vi "Build Tree from Section Change List.vi"(8 "error in (no error)":errorcluster, 9 "Database Changes":T1 {"Missing"."Node Ref" format="%.0x"; "Changed"."Old"."Node Ref" format="%.0x"}, 10 "Section":string="Incoming", 11 "TreeControl in":refnum<vi>) -> (0 "error out":errorcluster, 3 "TreeControl out":refnum<vi>)   [LabVIEW 2025, in "Protection and Counter Addon System Explorer.lvlib"]
uses:
  Protection and Counter Addon System Explorer.lvlib
  Types/Database Changes.ctl
  Types/Base Frame Info_NoVS.ctl
  Types/Signal Attributes.ctl
  Types/CAN Filter Type.ctl
  Types/Base Frame Info.ctl
  <vilib>/NI VeriStand/Custom Device API/Custom Device Item Ref.ctl
  Types/Related CAN Frames.ctl
  Types/Related CAN Frames No VS.ctl
  Types/Tree Item Settings.ctl
  <vilib>/NI VeriStand/Custom Device API/Custom Device API.lvlib
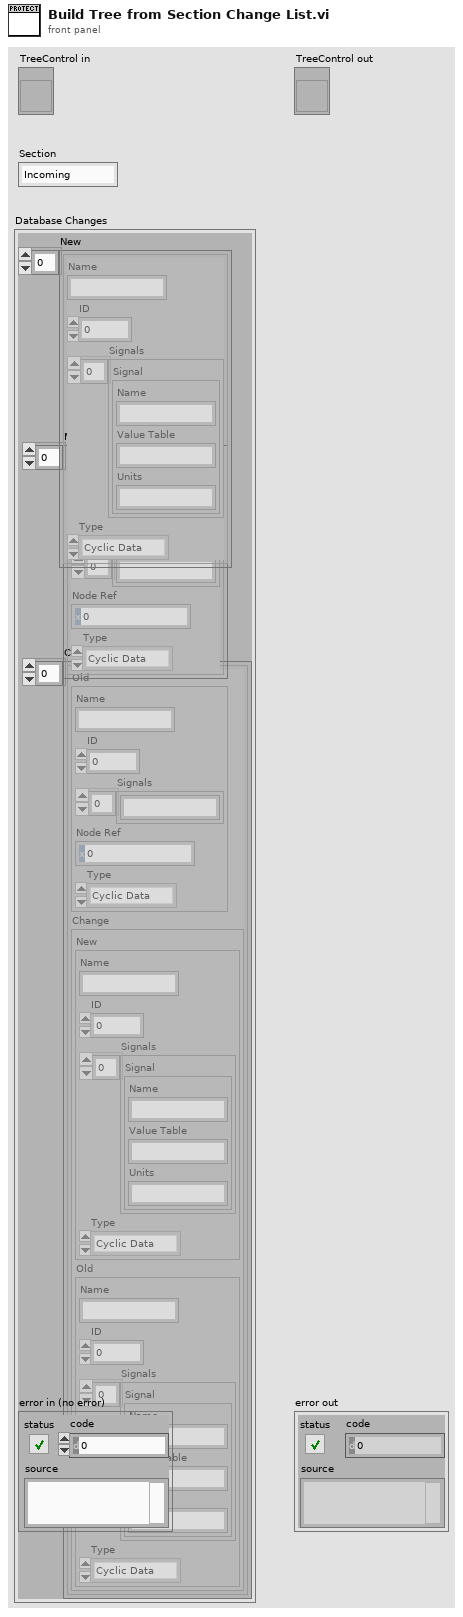
[diagram p1: front panel]
types:
  T1 = typedef "Protection and Counter Addon System Explorer.lvlib/Database Changes.ctl" = cluster{"New":T2[], "Missing":T5[], "Changed":T7[]}
  T2 = typedef "Protection and Counter Addon System Explorer.lvlib/Base Frame Info_NoVS.ctl" = cluster{"Name":string, "ID":u32, "Signals":T3[], "Type":T4}
  T3 = typedef "Protection and Counter Addon System Explorer.lvlib/Signal Attributes.ctl" = cluster{"Name":string, "Value Table":string, "Units":string}
  T4 = typedef "Protection and Counter Addon System Explorer.lvlib/CAN Filter Type.ctl" = enum16{"Cyclic Data", "Event Data", "Cyclic/Event", "All"}
  T5 = typedef "Protection and Counter Addon System Explorer.lvlib/Base Frame Info.ctl" = cluster{"Name":string, "ID":u32, "Signals":string[], "Node Ref":T6, "Type":T4}
  T6 = typedef "Custom Device API.lvlib/Custom Device Item Ref.ctl" = u64
  T7 = typedef "Protection and Counter Addon System Explorer.lvlib/Related CAN Frames.ctl" = cluster{"Old":T5, "Change":T8}
  T8 = typedef "Protection and Counter Addon System Explorer.lvlib/Related CAN Frames No VS.ctl" = cluster{"New":T2, "Old":T2}
  T9 = typedef "Protection and Counter Addon System Explorer.lvlib/Tree Item Settings.ctl" = cluster{"Name":string, "Background Color":u32, "Symbol":i32, "ChildText":string, "Disable":bool}
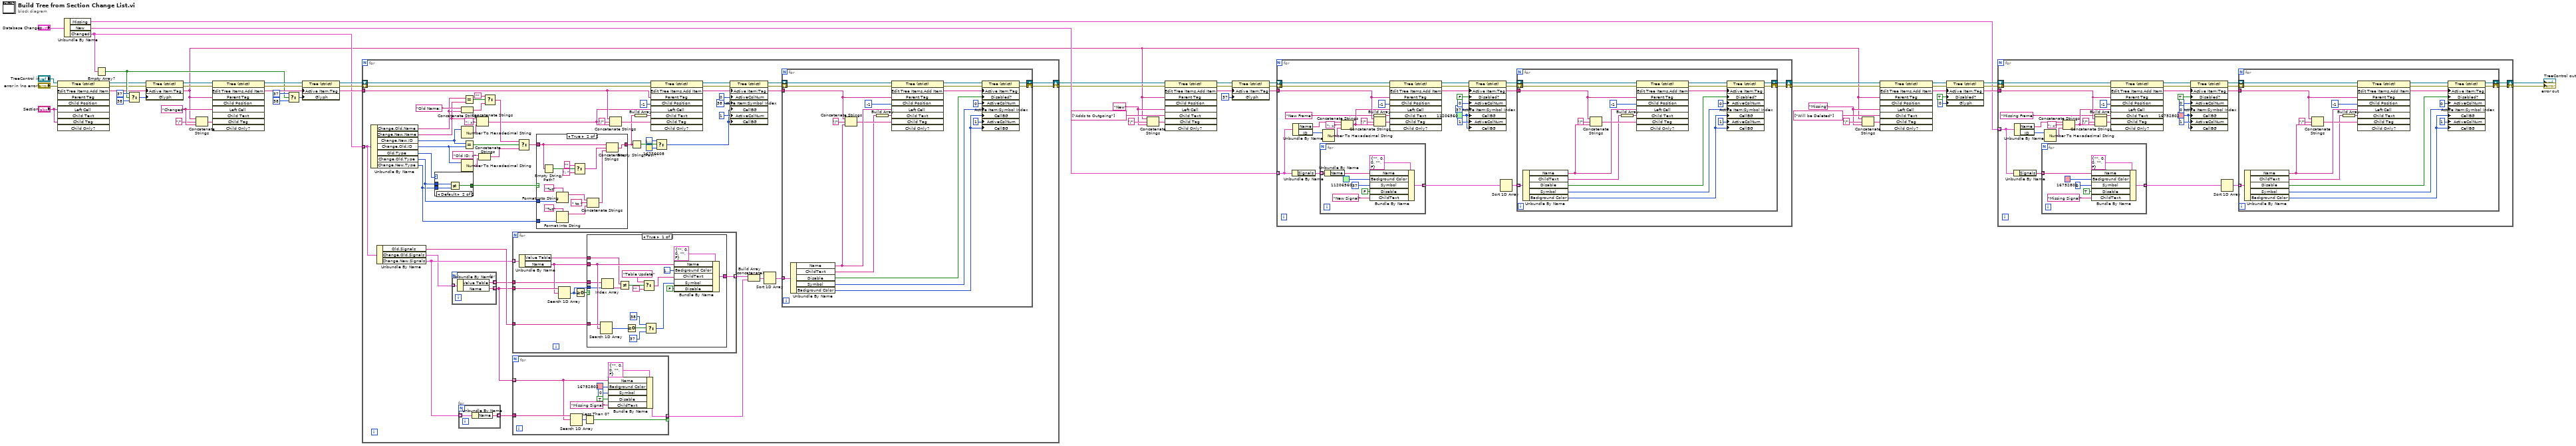
[diagram p0: block diagram]
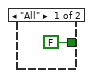
[diagram p2: hidden frame]
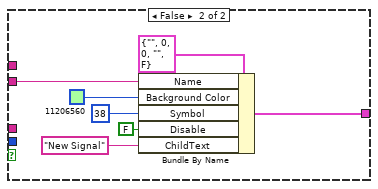
[diagram p4: hidden frame]
diagram:
  w3 = "Missing" ("Parent Tag")
  w6 = "New" ("Parent Tag")
  w22 = "Changed" ("Parent Tag")
  n1 = invoke on="Invoke Node" class="Tree (strict)" method="Edit Tree Items.Add Item"(reference="TreeControl in", error in="error in (no error)", "Left Cell"="Section", "Child Tag"="Section") -> (reference out=w11:refnum<vi>, error out=w9:errorcluster, "Edit Tree Items:Add Item"=w2:string)  [unwired: 5 in, 6 out]
  n2 = Unbundle By Name("Database Changes") -> ("Missing"=w35:T5[], "New"=w30:T2[], "Changed"=w19:T7[])
  n3 = Empty Array?(array=w19) -> (empty?=w12:bool)
  n4 = Select(t=37 ("Active Item:Symbol Index"), s=w12, f=38 ("Active Item:Symbol Index")) -> (s? t:f=w14:i32)
  n5 = property class="Tree (strict)"(reference=w11, error in=w9, "Active Item:Tag"=w2, "Glyph"=w14) -> (reference out=w10:refnum<vi>, error out=w8:errorcluster)
  n6 = Concatenate Strings(w2, "/" ("string"), w22) -> (w20:string)
  n7 = invoke on="Invoke Node" class="Tree (strict)" method="Edit Tree Items.Add Item"(reference=w10, error in=w8, "Parent Tag"=w2, "Left Cell"=w22, "Child Tag"=w20) -> (reference out=w37:refnum<vi>, error out=w38:errorcluster, "Edit Tree Items:Add Item"=w41:string)  [unwired: 4 in, 6 out]
  n8 = Select(t=37 ("Active Item:Symbol Index"), s=w12, f=38 ("Active Item:Symbol Index")) -> (s? t:f=w17:i32)
  n9 = property class="Tree (strict)"(reference=w37, error in=w38, "Active Item:Tag"=w41, "Glyph"=w17) -> (reference out=w40:refnum<vi>, error out=w39:errorcluster)
  n10 = for {
    tunnel: w19 -> [w80] mode=indexing
    shift-right: [w72] -> w28
    shift-left: w39 -> [w89]
    shift-right: [w71] -> w29
    shift-left: w40 -> [w105]
    tunnel: w41 -> [w68]
    n11 = Unbundle By Name(w80) -> ("Change.Old.Name"=w95:string, "Change.New.Name"=w99:string, "Change.New.ID"=w97:u32, "Change.Old.ID"=w101:u32, "Old.Type"=w60:T4, "Change.Old.Type"=w65:T4, "Change.New.Type"=w61:T4)
    n12 = Unbundle By Name(w80) -> ("Old.Signals"=w79:string[], "Change.Old.Signals"=w55:T3[], "Change.New.Signals"=w58:T3[])
    n13 = case shown="Default" w60 {
      tunnel: w65 -> [_ w117]
      tunnel: [FALSE w116] -> w64
      tunnel: w61 -> [_ w115]
      frame "All" {
      }
      frame Default {
        n14 = Not Equal?(x=w117, y=w115) -> (x != y?=w116:bool)
      }
    }
    n15 = for {
      tunnel: w55 -> [w111] mode=indexing
      tunnel: [w110] -> w59 mode=indexing
      tunnel: [w109] -> w56 mode=indexing
      n16 = Unbundle By Name(w111) -> ("Value Table"=w109:string, "Name"=w110:string)
    }
    n17 = for {
      tunnel: w58 -> [w113] mode=indexing
      tunnel: [w112] -> w57 mode=indexing
      n18 = Unbundle By Name(w113) -> ("Name"=w112:string)
    }
    n19 = Concatenate Strings("Old Name: ", w95) -> (w90:string)
    n20 = Number To Hexadecimal String(2:w97) -> (0:w96:string)  [unwired: 1 in]
    n21 = Number To Hexadecimal String(2:w101) -> (0:w100:string)  [unwired: 1 in]
    n22 = Equal?(x=w95, y=w99) -> (x = y?=w91:bool)
    n23 = Equal?(x=w97, y=w101) -> (x = y?=w94:bool)
    n24 = Concatenate Strings(w99, ": x" ("string"), w96) -> (w67:string)
    n25 = Concatenate Strings("Old ID: x", w100) -> (w93:string)
    n26 = Select(t="", s=w91, f=w90) -> (s? t:f=w87:string)
    n27 = for {
      tunnel: w59 -> [w171]
      tunnel: w58 -> [w169] mode=indexing
      tunnel: [w170] -> w78 mode=indexing
      tunnel: w79 -> [w166]
      tunnel: w56 -> [w163]
      n28 = Unbundle By Name(w169) -> ("Value Table"=w165:string, "Name"=w167:string)
      n29 = Search 1D Array(1D array=w171, element=w167) -> (index of element=w164:i32)  [unwired: 1 in]
      n30 = Greater Or Equal To 0?(x=w164) -> (x >= 0?=w168:bool)
      n31 = case shown="True" w168 {
        tunnel: [w184 w195] -> w170
        tunnel: w167 -> [w180 w191]
        tunnel: w166 -> [w182 _]
        tunnel: w165 -> [w176 _]
        tunnel: w164 -> [w178 _]
        tunnel: w163 -> [w179 _]
        frame True {
          n32 = Search 1D Array(1D array=w182, element=w180) -> (index of element=w183:i32)  [unwired: 1 in]
          n33 = Index Array(array=w179, index=w178) -> (element=w177:string)
          n34 = Not Equal?(x=w176, y=w177) -> (x != y?=w175:bool)
          n35 = Greater Or Equal To 0?(x=w183) -> (x >= 0?=w181:bool)
          n36 = Select(t="Table Update", s=w175, f="") -> (s? t:f=w172:string)
          n37 = Select(t=38 ("Active Item:Symbol Index"), s=w181, f=37 ("Active Item:Symbol Index")) -> (s? t:f=w187:i32)
          n38 = Bundle By Name(cluster=T9 {"Name"="", "Background Color"=0, "Symbol"=0, "ChildText"="", "Disable"=FALSE}, "Name"=w180, "Background Color"=u32 16777216, "ChildText"=w172, "Symbol"=w187, "Disable"=FALSE) -> (w184:T9)
        }
        frame False {
          n39 = Bundle By Name(cluster=T9 {"Name"="", "Background Color"=0, "Symbol"=0, "ChildText"="", "Disable"=FALSE}, "Name"=w191, "Background Color"=u32 11206560, "Symbol"=38 ("Active Item:Symbol Index"), "Disable"=FALSE, "ChildText"="New Signal" ("string")) -> (w195:T9)
        }
      }
    }
    n40 = for {
      tunnel: w57 -> [w162]
      tunnel: w59 -> [w153] mode=indexing
      tunnel: [w157] -> w77 mode=indexing if=w160
      n41 = Search 1D Array(1D array=w162, element=w153) -> (index of element=w161:i32)  [unwired: 1 in]
      n42 = Less Than 0?(x=w161) -> (x < 0?=w160:bool)
      n43 = Bundle By Name(cluster=T9 {"Name"="", "Background Color"=0, "Symbol"=0, "ChildText"="", "Disable"=FALSE}, "Name"=w153, "Background Color"=u32 16752802, "Symbol"=0 ("Active Item:Symbol Index"), "Disable"=TRUE, "ChildText"="Missing Signal" ("string")) -> (w157:T9)
    }
    n44 = Select(t=w87, s=w94, f=w93) -> (s? t:f=w63:string)
    n45 = case shown="True" w64 {
      tunnel: w65 -> [_ w132]
      tunnel: [w118 w130] -> w62
      tunnel: w63 -> [w118 w119]
      tunnel: w61 -> [_ w124]
      frame False {
      }
      frame True {
        n46 = Empty String/Path?(string/path=w119) -> (empty?=w129:bool)
        n47 = Format Into String(format string="%s", w132) -> (resulting string=w123:string)  [unwired: 2 in, 1 out]
        n48 = Format Into String(format string="%s", w124) -> (resulting string=w121:string)  [unwired: 2 in, 1 out]
        n49 = Select(t="", s=w129, f="; ") -> (s? t:f=w127:string)
        n50 = Concatenate Strings(w123, " to " ("string"), w121) -> (w120:string)
        n51 = Concatenate Strings(w119, w127, w120) -> (w130:string)
      }
    }
    n52 = Concatenate Strings(w68, "/" ("string"), w67) -> (w66:string)
    n53 = Empty String/Path?(string/path=w62) -> (empty?=w86:bool)
    n54 = Build Array(w62) -> (w88:string[])
    n55 = invoke on="Invoke Node" class="Tree (strict)" method="Edit Tree Items.Add Item"(reference=w105, error in=w89, "Parent Tag"=w68, "Child Position"=-1, "Left Cell"=w67, "Child Text"=w88, "Child Tag"=w66) -> (reference out=w108:refnum<vi>, error out=w107:errorcluster, "Edit Tree Items:Add Item"=w70:string)  [unwired: 2 in, 6 out]
    n56 = Select(t=u32 16777216, s=w86, f=u32 16776608) -> (s? t:f=w81:u32)
    n57 = property class="Tree (strict)"(reference=w108, error in=w107, "Active Item:Tag"=w70, "ActiveColNum"=0 ("Active Cell:Active Column Number"), "Active Item:Symbol Index"=38, "CellBG"=w81, "ActiveColNum"=1 ("Active Cell:Active Column Number"), "CellBG"=w81) -> (reference out=w75:refnum<vi>, error out=w74:errorcluster)
    n58 = Build Array (concatenate)(w78, w77) -> (w76:T9[])
    n59 = Sort 1D Array(array=w76) -> (sorted array=w73:T9[])
    n60 = for {
      shift-right: [w137] -> w71
      shift-left: w75 -> [w150]
      shift-right: [w138] -> w72
      shift-left: w74 -> [w136]
      tunnel: w73 -> [w148] mode=indexing
      tunnel: w70 -> [w149]
      n61 = Unbundle By Name(w148) -> ("Name"=w147:string, "ChildText"=w135:string, "Disable"=w134:bool, "Symbol"=w139:i32, "Background Color"=w133:u32)
      n62 = Concatenate Strings(w149, "/" ("string"), w147) -> (w146:string)
      n63 = Build Array(w135) -> (w145:string[])
      n64 = invoke on="Invoke Node" class="Tree (strict)" method="Edit Tree Items.Add Item"(reference=w150, error in=w136, "Parent Tag"=w149, "Child Position"=-1, "Left Cell"=w147, "Child Text"=w145, "Child Tag"=w146) -> (reference out=w142:refnum<vi>, error out=w141:errorcluster, "Edit Tree Items:Add Item"=w140:string)  [unwired: 2 in, 6 out]
      n65 = property class="Tree (strict)"(reference=w142, error in=w141, "Active Item:Tag"=w140, "Disabled?"=w134, "ActiveColNum"=0 ("Active Cell:Active Column Number"), "Active Item:Symbol Index"=w139, "CellBG"=w133, "ActiveColNum"=1 ("Active Cell:Active Column Number"), "CellBG"=w133) -> (reference out=w137:refnum<vi>, error out=w138:errorcluster)
    }
  }
  n66 = Concatenate Strings(w2, "/" ("string"), w6) -> (w5:string)
  n67 = invoke on="Invoke Node" class="Tree (strict)" method="Edit Tree Items.Add Item"(reference=w29, error in=w28, "Parent Tag"=w2, "Left Cell"=w6, "Child Text"=string[] ["Adds to Outgoing"], "Child Tag"=w5) -> (reference out=w44:refnum<vi>, error out=w45:errorcluster, "Edit Tree Items:Add Item"=w43:string)  [unwired: 3 in, 6 out]
  n68 = property class="Tree (strict)"(reference=w44, error in=w45, "Active Item:Tag"=w43, "Glyph"=37 ("Active Item:Symbol Index")) -> (reference out=w47:refnum<vi>, error out=w46:errorcluster)
  n69 = for {
    tunnel: w30 -> [w213] mode=indexing
    shift-right: [w208] -> w32
    shift-left: w46 -> [w217]
    shift-right: [w207] -> w31
    shift-left: w47 -> [w223]
    tunnel: w43 -> [w204]
    w200 = u32 11206560
    n70 = Unbundle By Name(w213) -> ("Signals"=w212:T3[])
    n71 = Unbundle By Name(w213) -> ("Name"=w221:string, "ID"=w219:u32)
    n72 = for {
      tunnel: w212 -> [w251] mode=indexing
      tunnel: [w252] -> w199 mode=indexing
      n73 = Unbundle By Name(w251) -> ("Name"=w247:string)
      n74 = Bundle By Name(cluster=T9 {"Name"="", "Background Color"=0, "Symbol"=0, "ChildText"="", "Disable"=FALSE}, "Name"=w247, "Background Color"=u32 11206560, "Symbol"=37 ("Active Item:Symbol Index"), "Disable"=FALSE, "ChildText"="New Signal" ("string")) -> (w252:T9)
    }
    n75 = Number To Hexadecimal String(2:w219) -> (0:w218:string)  [unwired: 1 in]
    n76 = Concatenate Strings(w221, ": x" ("string"), w218) -> (w203:string)
    n77 = Build Array("New Frame" ("string")) -> (w216:string[])
    n78 = Concatenate Strings(w204, "/" ("string"), w203) -> (w202:string)
    n79 = invoke on="Invoke Node" class="Tree (strict)" method="Edit Tree Items.Add Item"(reference=w223, error in=w217, "Parent Tag"=w204, "Child Position"=-1, "Left Cell"=w203, "Child Text"=w216, "Child Tag"=w202) -> (reference out=w226:refnum<vi>, error out=w225:errorcluster, "Edit Tree Items:Add Item"=w206:string)  [unwired: 2 in, 6 out]
    n80 = property class="Tree (strict)"(reference=w226, error in=w225, "Active Item:Tag"=w206, "Disabled?"=FALSE ("Active Item:Disabled?"), "ActiveColNum"=0 ("Active Cell:Active Column Number"), "Active Item:Symbol Index"=37, "CellBG"=w200, "ActiveColNum"=1 ("Active Cell:Active Column Number"), "CellBG"=w200) -> (reference out=w211:refnum<vi>, error out=w210:errorcluster)
    n81 = Sort 1D Array(array=w199) -> (sorted array=w209:T9[])
    n82 = for {
      shift-right: [w231] -> w207
      shift-left: w211 -> [w244]
      shift-right: [w232] -> w208
      shift-left: w210 -> [w230]
      tunnel: w209 -> [w242] mode=indexing
      tunnel: w206 -> [w243]
      n83 = Unbundle By Name(w242) -> ("Name"=w241:string, "ChildText"=w229:string, "Disable"=w228:bool, "Symbol"=w233:i32, "Background Color"=w227:u32)
      n84 = Concatenate Strings(w243, "/" ("string"), w241) -> (w240:string)
      n85 = Build Array(w229) -> (w239:string[])
      n86 = invoke on="Invoke Node" class="Tree (strict)" method="Edit Tree Items.Add Item"(reference=w244, error in=w230, "Parent Tag"=w243, "Child Position"=-1, "Left Cell"=w241, "Child Text"=w239, "Child Tag"=w240) -> (reference out=w236:refnum<vi>, error out=w235:errorcluster, "Edit Tree Items:Add Item"=w234:string)  [unwired: 2 in, 6 out]
      n87 = property class="Tree (strict)"(reference=w236, error in=w235, "Active Item:Tag"=w234, "Disabled?"=w228, "ActiveColNum"=0 ("Active Cell:Active Column Number"), "Active Item:Symbol Index"=w233, "CellBG"=w227, "ActiveColNum"=1 ("Active Cell:Active Column Number"), "CellBG"=w227) -> (reference out=w231:refnum<vi>, error out=w232:errorcluster)
    }
  }
  n88 = Concatenate Strings(w2, "/" ("string"), w3) -> (w1:string)
  n89 = invoke on="Invoke Node" class="Tree (strict)" method="Edit Tree Items.Add Item"(reference=w31, error in=w32, "Parent Tag"=w2, "Left Cell"=w3, "Child Text"=string[] ["Will be Deleted"], "Child Tag"=w1) -> (reference out=w52:refnum<vi>, error out=w50:errorcluster, "Edit Tree Items:Add Item"=w54:string)  [unwired: 3 in, 6 out]
  n90 = property class="Tree (strict)"(reference=w52, error in=w50, "Active Item:Tag"=w54, "Disabled?"=TRUE ("Active Item:Disabled?"), "Glyph"=0 ("Active Item:Symbol Index")) -> (reference out=w53:refnum<vi>, error out=w51:errorcluster)
  n91 = for {
    tunnel: w35 -> [w270] mode=indexing
    shift-right: [w265] -> w34
    shift-left: w51 -> [w274]
    shift-right: [w264] -> w33
    shift-left: w53 -> [w280]
    tunnel: w54 -> [w261]
    w257 = u32 16752802
    n92 = Unbundle By Name(w270) -> ("Signals"=w269:string[])
    n93 = Unbundle By Name(w270) -> ("Name"=w278:string, "ID"=w276:u32)
    n94 = for {
      tunnel: w269 -> [w307] mode=indexing
      tunnel: [w308] -> w256 mode=indexing
      n95 = Bundle By Name(cluster=T9 {"Name"="", "Background Color"=0, "Symbol"=0, "ChildText"="", "Disable"=FALSE}, "Name"=w307, "Background Color"=u32 16752802, "Symbol"=0 ("Active Item:Symbol Index"), "Disable"=TRUE, "ChildText"="Missing Signal" ("string")) -> (w308:T9)
    }
    n96 = Number To Hexadecimal String(2:w276) -> (0:w275:string)  [unwired: 1 in]
    n97 = Concatenate Strings(w278, ": x" ("string"), w275) -> (w260:string)
    n98 = Build Array("Missing Frame" ("string")) -> (w273:string[])
    n99 = Concatenate Strings(w261, "/" ("string"), w260) -> (w259:string)
    n100 = invoke on="Invoke Node" class="Tree (strict)" method="Edit Tree Items.Add Item"(reference=w280, error in=w274, "Parent Tag"=w261, "Child Position"=-1, "Left Cell"=w260, "Child Text"=w273, "Child Tag"=w259) -> (reference out=w283:refnum<vi>, error out=w282:errorcluster, "Edit Tree Items:Add Item"=w263:string)  [unwired: 2 in, 6 out]
    n101 = property class="Tree (strict)"(reference=w283, error in=w282, "Active Item:Tag"=w263, "Disabled?"=TRUE ("Active Item:Disabled?"), "ActiveColNum"=0 ("Active Cell:Active Column Number"), "Active Item:Symbol Index"=0, "CellBG"=w257, "ActiveColNum"=1 ("Active Cell:Active Column Number"), "CellBG"=w257) -> (reference out=w268:refnum<vi>, error out=w267:errorcluster)
    n102 = Sort 1D Array(array=w256) -> (sorted array=w266:T9[])
    n103 = for {
      shift-right: [w288] -> w264
      shift-left: w268 -> [w301]
      shift-right: [w289] -> w265
      shift-left: w267 -> [w287]
      tunnel: w266 -> [w299] mode=indexing
      tunnel: w263 -> [w300]
      n104 = Unbundle By Name(w299) -> ("Name"=w298:string, "ChildText"=w286:string, "Disable"=w285:bool, "Symbol"=w290:i32, "Background Color"=w284:u32)
      n105 = Concatenate Strings(w300, "/" ("string"), w298) -> (w297:string)
      n106 = Build Array(w286) -> (w296:string[])
      n107 = invoke on="Invoke Node" class="Tree (strict)" method="Edit Tree Items.Add Item"(reference=w301, error in=w287, "Parent Tag"=w300, "Child Position"=-1, "Left Cell"=w298, "Child Text"=w296, "Child Tag"=w297) -> (reference out=w293:refnum<vi>, error out=w292:errorcluster, "Edit Tree Items:Add Item"=w291:string)  [unwired: 2 in, 6 out]
      n108 = property class="Tree (strict)"(reference=w293, error in=w292, "Active Item:Tag"=w291, "Disabled?"=w285, "ActiveColNum"=0 ("Active Cell:Active Column Number"), "Active Item:Symbol Index"=w290, "CellBG"=w284, "ActiveColNum"=1 ("Active Cell:Active Column Number"), "CellBG"=w284) -> (reference out=w288:refnum<vi>, error out=w289:errorcluster)
    }
  }
  "error out" <- w34
  "TreeControl out" <- w33
